vi "Start Bus Monitor.vi"(8 "error in (no error)":errorcluster, 10 "MediatorBusMonitor (Type)":refnum<class "IMediatorBusMonitor.lvclass">, 11 "IMediator In":refnum<class "IMediator.lvclass">) -> (0 "error out":errorcluster, 3 "IMediator Out":refnum<class "IMediator.lvclass">)   [LabVIEW 2015, in "IMediator.lvlib" / "IMediator.lvclass"]
uses:
  IMediator.lvclass
  IMediatorBusMonitor/MediatorBusMonitor/IMediatorBusMonitor.lvclass
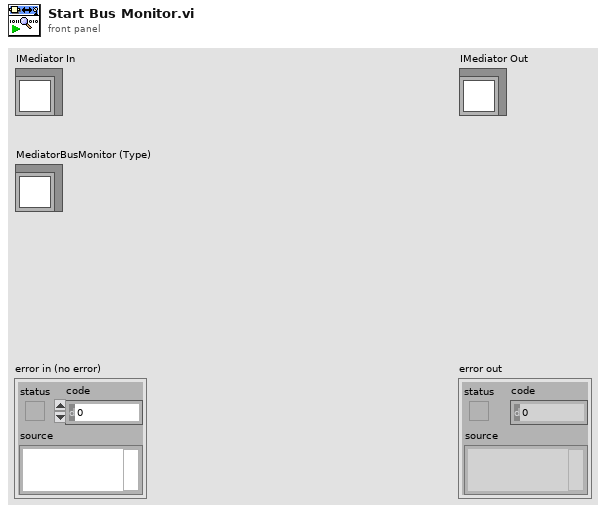
[diagram p1: front panel]
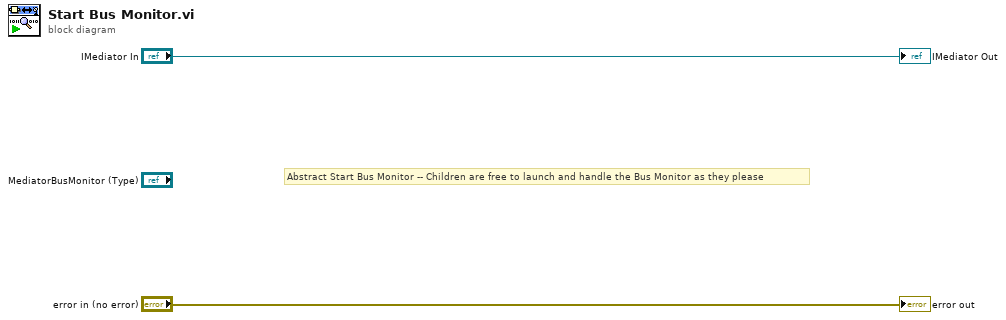
[diagram p0: block diagram]
diagram:
  # "Abstract Start Bus Monitor -- Children are free to launch and handle the Bus Monitor as they please"
  "error out" <- "error in (no error)"
  "IMediator Out" <- "IMediator In"
